vi "Do.vi"(8 "Error In":errorcluster, 10 "Actor in":refnum<class "Actor.lvclass">, 11 "LNA Connection Status Msg":refnum<class "LNA Connection Status Msg.lvclass">) -> (0 "Error Out":errorcluster, 2 "Actor out":refnum<class "Actor.lvclass">)   [LabVIEW 2014, in "CS++RTMain.lvlib" / "LNA Connection Status Msg.lvclass"]
doc: "(<B>Filename</B>: Actor Framework.lvlib:Message.lvclass:Do.vi)\n\nDefines what a message does when it is received by an actor. Generally, a message instructs an actor to invoke one of its methods. By default, this method does nothing. A child class must override it to define behavior. Create a child class by using the Actor Framework Message Maker dialog box."
uses:
  LNA Connection Status Msg.lvclass
  <vilib>/ActorFramework/Actor/Actor.lvclass
  <vilib>/NI/Actors/Linked Network Actor/Linked Network Actor Messages/LNA Connection Status Msg/LNA Connection Status Msg.lvclass/LNA Connection Status Msg.ctl
  CS++RTMain/CS++RTMainActor.lvclass
  CS++RTMain/CS++RTMainActor.lvclass/CS++RTMainActor.ctl
  <vilib>/NI/Actors/Linked Network Actor/Linked Network Actor Messages/LNA Connection Status Msg/LNA Connection Status Msg.lvclass
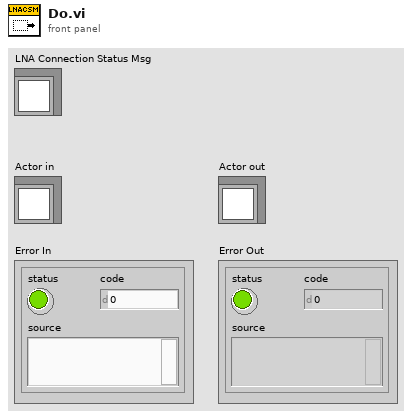
[diagram p1: front panel]
types:
  T1 = cluster{"Name":string, "Writer":bool, "Reader":bool}
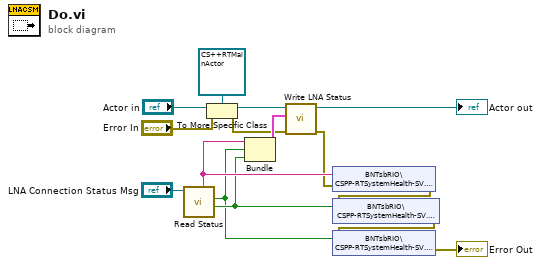
[diagram p0: block diagram]
diagram:
  n1 = call <vilib>:"Read Status.vi"("Update Status Msg in"="LNA Connection Status Msg") -> ("Reader"=w11:bool, "Writer"=w10:bool, "Name"=w12:string)  [unwired: 7 in, 1 out]
  n2 = To More Specific Class(target class=refnum<class "CS++RTMainActor.lvclass"> refnum ("CS++RTMain.lvlib:CS++RTMainActor.lvclass"), reference="Actor in", error in="Error In") -> (specific class reference=w3:refnum<class "CS++RTMainActor.lvclass">, error out=w5:errorcluster)
  n3 = Bundle("Name"=w12, "Writer"=w10, "Reader"=w11) -> (w6:T1)  [unwired: 1 in]
  n4 = call "Write LNA Status.vi"("Error In"=w5, "LNA Status"=w6, "CS++RTMainActor in"=w3) -> ("Error Out"=w2:errorcluster, "CS++RTMainActor out"=→"Actor out":refnum<class "CS++RTMainActor.lvclass">)  [unwired: 7 in]
  n5 = shared-variable "BNTsbRIO\\CSPP-RTSystemHealth-SV.lvlib\\LNA Name"(w12, error in=w2) -> (error out=w9:errorcluster)
  n6 = shared-variable "BNTsbRIO\\CSPP-RTSystemHealth-SV.lvlib\\LNA Reader"(w11, error in=w9) -> (error out=w8:errorcluster)
  n7 = shared-variable "BNTsbRIO\\CSPP-RTSystemHealth-SV.lvlib\\LNA Writer"(w10, error in=w8) -> (error out=→"Error Out":errorcluster)
